vi "Stop Core.vi"(10 "final error code":i32, 11 "Person in":refnum<class "Person.lvclass">) -> (3 "Person out":refnum<class "Person.lvclass">)   [LabVIEW 2023, in "Person.lvlib" / "Person.lvclass"]
doc: "(<B>Filename</B>: Actor Framework.lvlib:Actor.lvclass:Stop Core.vi)\n\nDefines what the actor does before it stops. Use the <B>final error code</B> input to determine whether the actor shut down in response to an error.\n\nBy default, this method does nothing. A descendant class may override it to define behavior, such as shutting down any processes the actor initiated in its override of the Actor Core method."
uses:
  Person.lvclass
  Person.lvclass/Person.ctl
  <vilib>/ActorFramework/Actor/Actor.lvclass
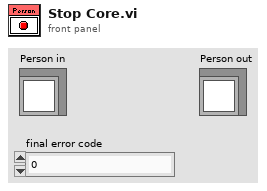
[diagram p1: front panel]
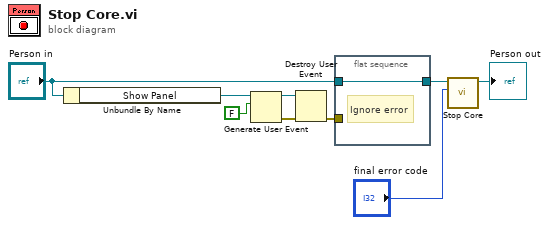
[diagram p0: block diagram]
diagram:
  n1 = Unbundle By Name("Person in") -> ("Show Panel"=w1:refnum<user-event>)
  n2 = Generate User Event(user event=w1, event data cluster=FALSE ("event data")) -> (user event out=w3:refnum<user-event>, error out=w4:errorcluster)  [unwired: 2 in]
  n3 = Destroy User Event(user event=w3, error in=w4) -> (error out=w2:errorcluster)
  n4 = flat-sequence {
    tunnel: "Person in" -> [w10]
    tunnel: [w10] -> w5
    tunnel: w2 -> [_]
    frame #0 {
      # "Ignore error"
    }
  }
  n5 = call-parent "Stop Core.vi"("final error code"="final error code", "Actor in"=w5) -> ("Actor out"=→"Person out":refnum<class "Person.lvclass">)  [unwired: 9 in]
